vi "AG33XXX.set GaussLL.vi"(2 "error in (no error)":errorcluster, 3 "i ref in":refnum<vi>, 4 "length [us]":dbl=0.02 format="%^#.3e", 5 "VISA in":refnum<visa-resource-name>="GPIB0::8::INSTR") -> (0 "error out":errorcluster, 1 "VISA out":refnum<visa-resource-name>)   [LabVIEW 2014, in "AG33XXX.lvlib"]
doc: "Low-level part of the Gaussian programming procedure. Included in this class since\nI did not want it to be confused with the VERY low-level stuff in the LabVIEW instr.lib.\n\nHistory: JULY-2004, Stefan Schwarz"
uses:
  AG33XXX.lvlib
  CSinstr.lib/Agilent 33xxx Series/Agilent 33XXX Series.lvlib
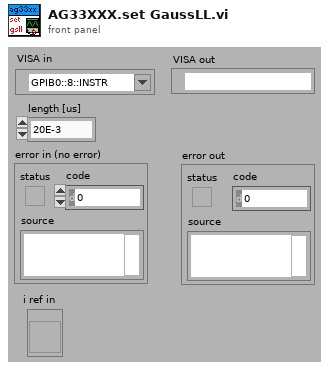
[diagram p1: front panel]
types:
  T1 = typedef "AG33XXX.lvlib/AG33XXX.i attribute.ctl" = cluster{"Gauss_Offset":dbl}
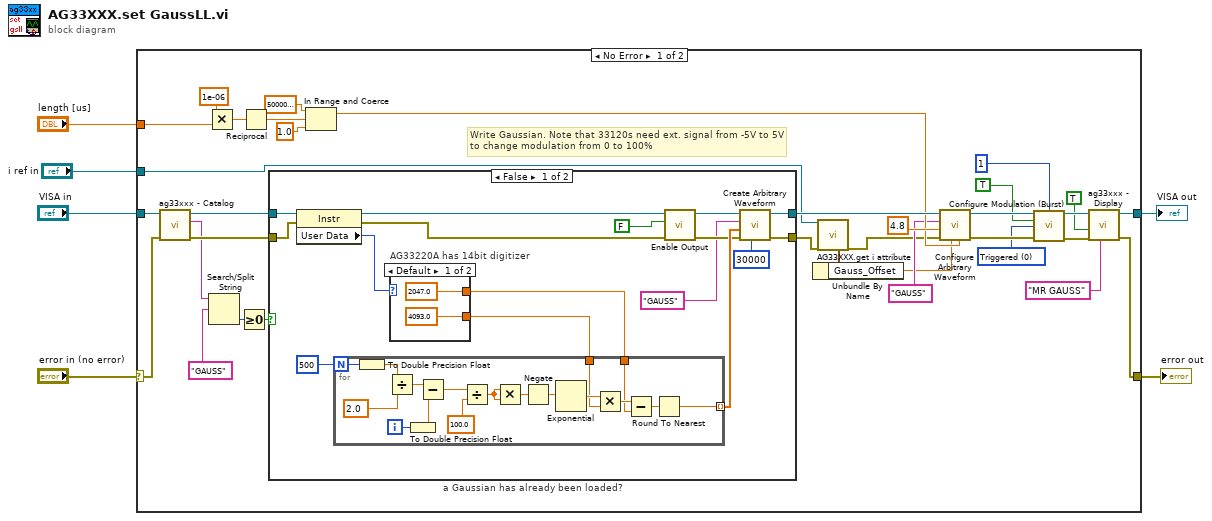
[diagram p0: block diagram]
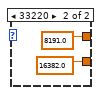
[diagram p2: hidden frame]
diagram:
  n1 = case shown="No Error" "error in (no error)" {
    selector: "error in (no error)" -> [w24 w80]
    tunnel: "length [us]" -> [w40 _]
    tunnel: "VISA in" -> [w25 w81]
    tunnel: [w14 w80] -> w4
    tunnel: [w16 w81] -> w3
    tunnel: "i ref in" -> [w11 _]
    frame No Error {
      w29 = u16 0 items=["Triggered", "Gated"] ("Burst Modulation Mode (0: Triggered)")
      # "Write Gaussian. Note that 33120s need ext. signal from -5V to 5V\nto change modulation from 0 to 100%"
      n2 = call "ag33xxx - Catalog.vi"("error in (no error)"=w24, "VISA session"=w25) -> ("error out"=w22:errorcluster, "Catalog"=w19:string, "dup VISA session"=w23:refnum<visa-resource-name>)  [unwired: 7 in]
      n3 = Multiply(x=1e-06 ("upper limit"), y=w40) -> (x*y=w32:dbl)
      n4 = Search/Split String(string=w19, search string/char (-)="GAUSS") -> (offset of match=w21:i32)  [unwired: 1 in, 2 out]
      n5 = Greater Or Equal To 0?(x=w21) -> (x >= 0?=w20:bool)
      n6 = Reciprocal(x=w32) -> (1/x=w39:dbl)
      n7 = case "a Gaussian has already been loaded?" shown="False" w20 {
        tunnel: [w51 w79] -> w35
        tunnel: [w50 w78] -> w10
        tunnel: w23 -> [w47 w79]
        tunnel: w22 -> [w46 w78]
        frame False {
          n8 = property class="Instr"(reference=w47, error in=w46) -> (reference out=w44:refnum<visa-resource-name>, error out=w45:errorcluster, "User Data"=w43:u32)
          n9 = case "AG33220A has 14bit digitizer" shown="Default" w43 {
            tunnel: [4093.0 ("y") 16382.0 ("y")] -> w42
            tunnel: [2047.0 ("y") 8191.0 ("y")] -> w41
            frame Default {
            }
            frame 33220 {
            }
          }
          n10 = for {
            N: 500 -> [w76]
            tunnel: [w63] -> w55 mode=indexing
            tunnel: w42 -> [w62]
            tunnel: w41 -> [w61]
            i -> [w77]
            n11 = To Double Precision Float(number=w76) -> (double precision float=w74:dbl)
            n12 = Divide(x=w74, y=2.0) -> (x/y=w73:dbl)
            n13 = To Double Precision Float(number=w77) -> (double precision float=w72:dbl)
            n14 = Subtract(x=w73, y=w72) -> (x-y=w71:dbl)
            n15 = Divide(x=w71, y=100.0) -> (x/y=w70:dbl)
            n16 = Multiply(x=w70, y=w70) -> (x*y=w69:dbl)
            n17 = Negate(x=w69) -> (-x=w68:dbl)
            n18 = Exponential(1:w68) -> (0:w67:dbl)
            n19 = Multiply(x=w67, y=w62) -> (x*y=w66:dbl)
            n20 = Subtract(x=w66, y=w61) -> (x-y=w65:dbl)
            n21 = Round To Nearest(number=w65) -> (nearest integer value=w63:dbl)
          }
          n22 = call "Enable Output.vi"("error in (no error)"=w45, "Enable Output (T: Enable)"=FALSE, "VISA resource name"=w44) -> ("error out"=w53:errorcluster, "VISA resource name out"=w54:refnum<visa-resource-name>)  [unwired: 7 in]
          n23 = call "Create Arbitrary Waveform.vi"("Timeout (10000)"=u32 30000, "error in (no error)"=w53, "Arbitrary Waveform Data"=w55, "Arbitrary Waveform Name (\"ARB1\")"="GAUSS", "VISA resource name"=w54) -> ("error out"=w50:errorcluster, "VISA resource name out"=w51:refnum<visa-resource-name>)  [unwired: 5 in]
        }
        frame True {
        }
      }
      n24 = In Range and Coerce(upper limit=5000000.0, x=w39, lower limit=1.0) -> (coerced(x)=w33:dbl)  [unwired: 1 out]
      n25 = call "AG33XXX.get i attribute.vi"("i ref in"=w11, "error in (no error)"=w10) -> ("i attribute"=w8:T1, "error out"=w9:errorcluster)  [unwired: 15 in, 1 out]
      n26 = Unbundle By Name(w8) -> ("Gauss_Offset"=w7:dbl)
      n27 = call "Configure Arbitrary Waveform.vi"("Frequency (1000 Hz)"=w33, "Offset (0.00 V)"=w7, "error in"=w9, "Gain (1.0)"=4.8, "Arbitrary Waveform Name (\"ARB1\")"="GAUSS", "VISA resource name"=w35) -> ("error out"=w30:errorcluster, "VISA resource name out"=w31:refnum<visa-resource-name>)  [unwired: 4 in]
      n28 = call "Configure Modulation (Burst).vi"("VISA resource name"=w31, "Burst Count (1)"=1, "Enable Burst Modulation (True)"=TRUE, "Burst Modulation Mode (0: Triggered)"=w29, "error in (no error)"=w30) -> ("VISA resource name out"=w17:refnum<visa-resource-name>, "error out"=w15:errorcluster)  [unwired: 9 in]
      n29 = call "ag33xxx - Display.vi"("Display Text"="MR GAUSS", "error in (no error)"=w15, "Text (F: off)"=TRUE, "VISA session"=w17) -> ("error out"=w14:errorcluster, "dup VISA session"=w16:refnum<visa-resource-name>)  [unwired: 6 in]
    }
    frame Error {
    }
  }
  "error out" <- w4
  "VISA out" <- w3
